vi "BuildHeaderData.vi"(5 "ScanFunc":i32, 6 "chemin Data":path, 8 "error in":errorcluster caption="entrée d'erreur (pas d'erreur)", 9 "SinglePar":bool, 10 "IndCourbe":i64, 11 "Experiment.lvclass In":refnum<class "Experiment.lvclass">) -> (0 "error out":errorcluster caption="sortie d'erreur", 1 "NomDon":string[](array[string])=["RTêta;", "X&Y;"], 2 "HeaderPar":string, 3 "Experiment.lvclass Out":refnum<class "Experiment.lvclass">, 4 "VarParams":string[][](array[string]), 7 "Experiment Name":string)   [LabVIEW 2019, in "Experiment.lvclass"]
uses:
  Experiment.lvclass
  Experiment.lvclass/Experiment.ctl
  DevicesClass/BaseDevice/BaseDevice.lvclass/BaseDevice.ctl
  DevicesClass/BaseDevice/Accessor/SetBaseDataPath.vi
  DevicesClass/BaseDevice/BaseDevice.lvclass
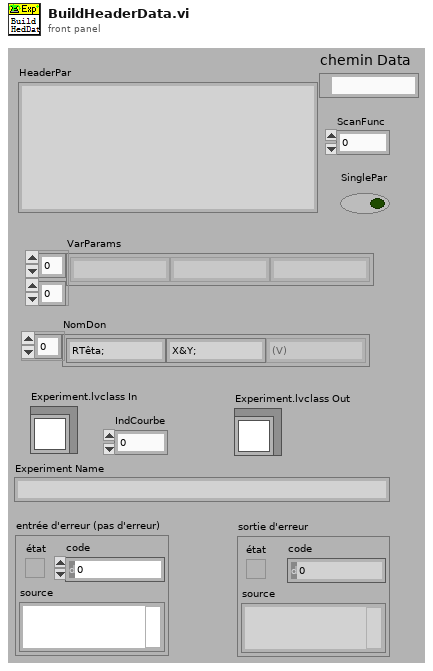
[diagram p1: front panel]
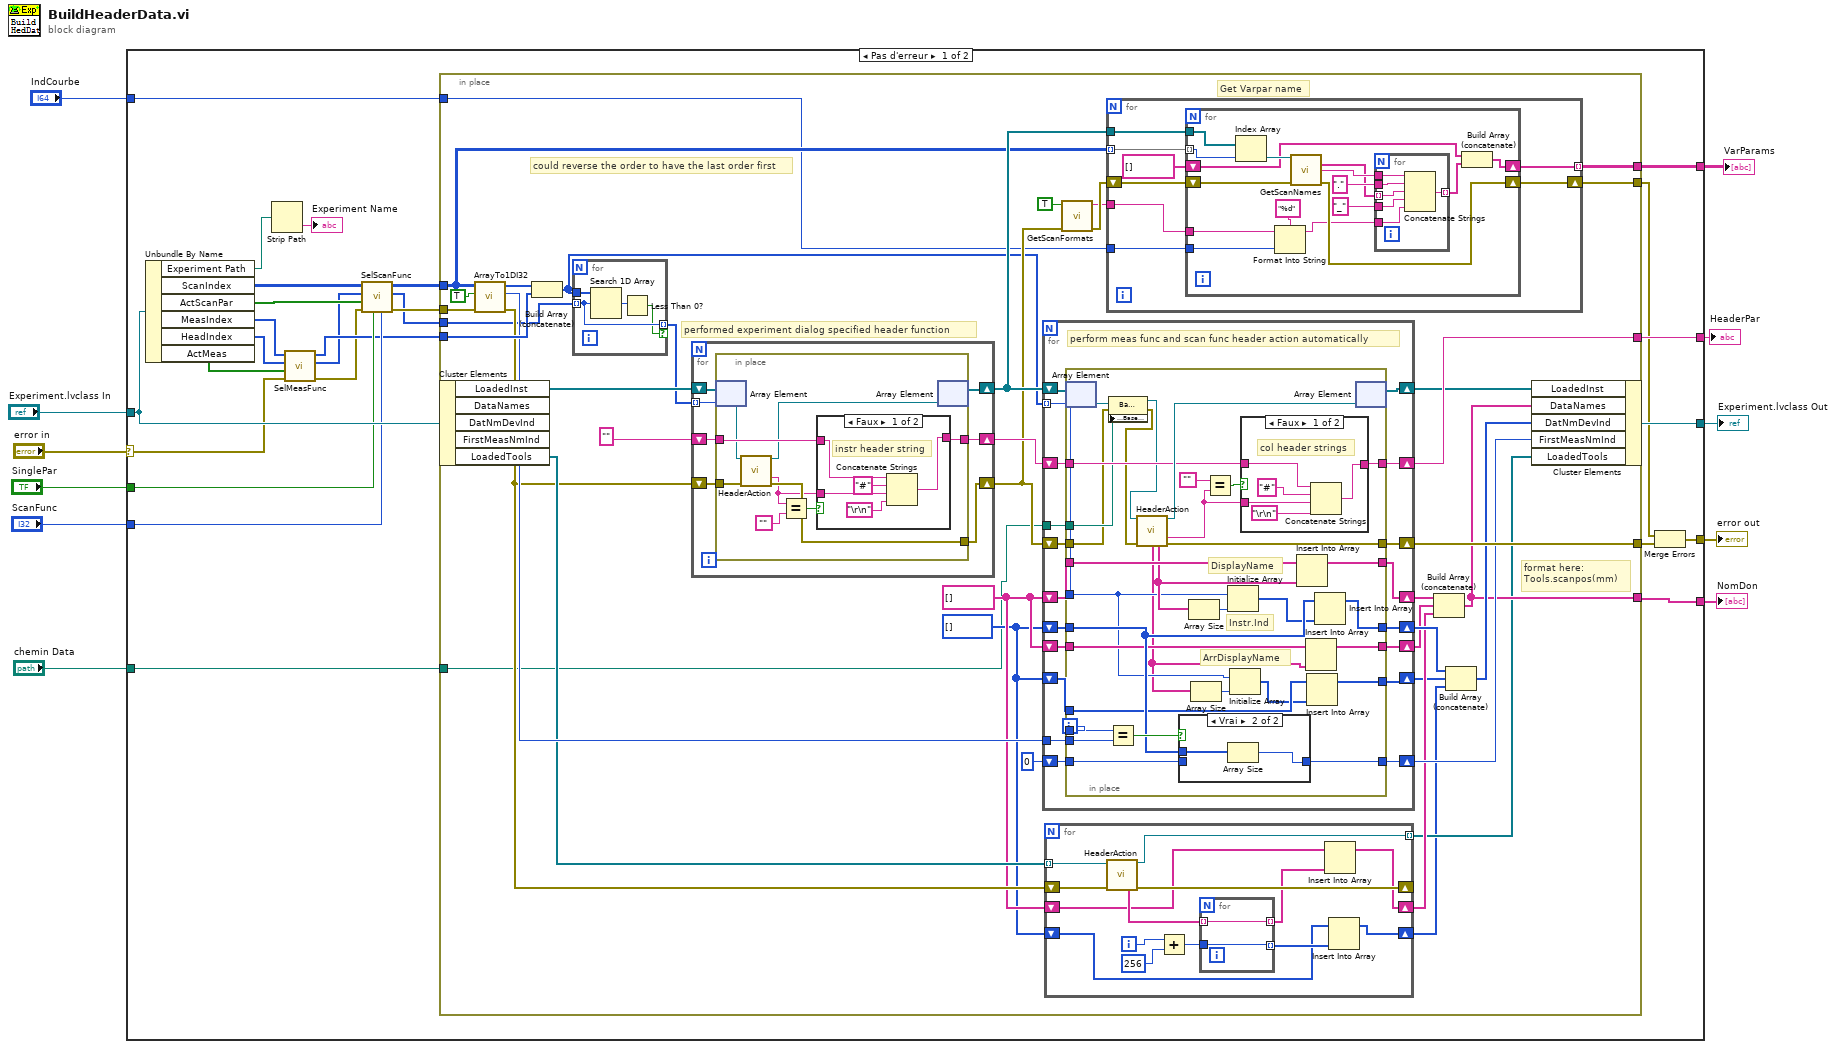
[diagram p0: block diagram]
diagram:
  n1 = case shown="Pas d'erreur" "error in" {
    selector: "error in" -> [w18 w211]
    tunnel: [w30 w211] -> w10
    tunnel: [w37 _] -> w9
    tunnel: [w33 _] -> w8
    tunnel: "Experiment.lvclass In" -> [w36 w210]
    tunnel: [w35 w210] -> w6
    tunnel: [w32 _] -> w5
    tunnel: "IndCourbe" -> [w31 _]
    tunnel: "SinglePar" -> [w20 _]
    tunnel: "ScanFunc" -> [w19 _]
    tunnel: "chemin Data" -> [w27 _]
    frame No Error {
      n2 = Unbundle By Name(w36) -> ("Experiment Path"=w21:path, "ScanIndex"=w23:i32[][], "ActScanPar"=w22:bool[], "MeasIndex"=w15:i32[], "HeadIndex"=w17:i32[], "ActMeas"=w14:bool[])
      n3 = Strip Path(path=w21) -> (name=→"Experiment Name":string)  [unwired: 1 out]
      n4 = call "SelMeasFunc.vi"("ErrorIn(No Error)"=w18, "Active MeasPar"=w14, "ScanHeaderIn"=w17, "MeasIndexIn"=w15) -> ("sortie d'erreur"=w13:errorcluster, "ScanHeaderOut"=w12:i32[], "MeasIndexOut"=w16:i32[])  [unwired: 5 in]
      n5 = call "SelScanFunc.vi"("Function"=w19, "SInglePar"=w20, "ErrorIn(No Error)"=w13, "Active ScanPar"=w22, "ScanHeaderIn"=w12, "ScanIndexIn"=w23) -> ("sortie d'erreur"=w26:errorcluster, "ScanHeaderOut"=w24:i32[], "ScanIndexOut"=w25:i32[][])  [unwired: 3 in]
      n6 = in-place {
        in-place-border: [w76] -> w37
        in-place-border: [w49] -> w33
        in-place-border: w26 -> [w71]
        in-place-border: w16 -> [w69]
        in-place-border: [w68] -> w34
        in-place-border: w25 -> [w61]
        in-place-border: w24 -> [w41]
        in-place-border: [w62] -> w32
        in-place-border: w31 -> [w56]
        in-place-border: [w55] -> w29
        in-place-border: w27 -> [w38]
        w45 = i32[] []
        w46 = string[] []
        # "format here:\nTools.scanpos(mm)"
        # "performed experiment dialog specified header function"
        # "Get Varpar name"
        # "could reverse the order to have the last order first"
        n7 = in-place-cluster #1(w36) -> ("LoadedInst"=w73:refnum<class "BaseDevice.lvclass">[], "LoadedTools"=w53:refnum<class "BaseDevice.lvclass">[])  [unwired: 3 out]
        n8 = call <userlib>:"ArrayTo1DI32.vi"("ErrorIn(No Error)"=w71, "DelArrEnd"=TRUE, "tableau"=w61) -> ("sortie d'erreur"=w52:errorcluster, "Size"=w66:i32, "Array Out"=w70:i32[])  [unwired: 6 in]
        n9 = Build Array (concatenate)(w70, w69) -> (w40:i32[])
        n10 = for {
          tunnel: w41 -> [w78] mode=indexing
          tunnel: w40 -> [w80]
          tunnel: [w78] -> w39 mode=indexing if=w77
          n11 = Search 1D Array(1D array=w80, element=w78) -> (index of element=w79:i32)  [unwired: 1 in]
          n12 = Less Than 0?(x=w79) -> (x < 0?=w77:bool)
        }
        n13 = for {
          shift-right: [w131] -> w74
          shift-left: "" -> [w132]
          tunnel: w39 -> [w130] mode=indexing
          shift-right: [w128] -> w63
          shift-left: w73 -> [w129]
          shift-right: [w127] -> w58
          shift-left: w52 -> [w133]
          n14 = in-place {
            in-place-border: w133 -> [w142]
            in-place-border: w132 -> [w141]
            in-place-border: [w138] -> w127
            in-place-border: [w136] -> w131
            n15 = in-place-array #2(w129, w130) -> (w135:refnum<class "BaseDevice.lvclass">)
            n16 = call-dynamic "HeaderAction.vi"("Device en entrée"=w135, "error in (no error)"=w142) -> ("Device en sortie"=w134:refnum<class "BaseDevice.lvclass">, "HeaderString"=w137:string, "error out"=w138:errorcluster)  [unwired: 7 in, 4 out]
            n17 = Equal?(x=w137, y="") -> (x = y?=w140:bool)
            n18 = case shown="Faux" w140 {
              tunnel: [w146 w148] -> w136
              tunnel: w137 -> [w144 _]
              tunnel: w141 -> [w145 w148]
              frame False {
                # "instr header string"
                n19 = Concatenate Strings(w145, "#" ("chaîne"), w144, "\r\n") -> (w146:string)
              }
              frame True {
              }
            }
            n20 = in-place-array #2(w134) -> (w128:refnum<class "BaseDevice.lvclass">[])  [unwired: 1 out]
          }
        }
        n21 = for {
          shift-right: [w167] -> w76
          shift-left: w74 -> [w164]
          shift-right: [w166] -> w50
          shift-left: w46 -> [w165]
          tunnel: w40 -> [w160] mode=indexing
          shift-right: [w162] -> w72
          shift-left: w63 -> [w163]
          shift-right: [w161] -> w68
          shift-left: w58 -> [w168]
          shift-right: [w159] -> w67
          shift-left: w45 -> [w158]
          tunnel: w66 -> [w157]
          shift-right: [w155] -> w64
          shift-left: 0 -> [w154]
          shift-right: [w153] -> w42
          shift-left: w46 -> [w152]
          shift-right: [w150] -> w43
          shift-left: w45 -> [w151]
          tunnel: w38 -> [w149]
          i -> [w156]
          # "perform meas func and scan func header action automatically"
          n22 = in-place {
            in-place-border: w168 -> [w170]
            in-place-border: [w200] -> w161
            in-place-border: [w199] -> w167
            in-place-border: [w198] -> w166
            in-place-border: w165 -> [w197]
            in-place-border: w164 -> [w192]
            in-place-border: w160 -> [w177]
            in-place-border: [w190] -> w159
            in-place-border: w158 -> [w186]
            in-place-border: w157 -> [w188]
            in-place-border: w156 -> [w189]
            in-place-border: [w185] -> w155
            in-place-border: w154 -> [w184]
            in-place-border: [w179] -> w153
            in-place-border: w152 -> [w178]
            in-place-border: w151 -> [w176]
            in-place-border: [w174] -> w150
            in-place-border: w149 -> [w172]
            # "ArrDisplayName"
            # "Instr.Ind"
            # "DisplayName"
            n23 = in-place-array #3(w163, w160) -> (w191:refnum<class "BaseDevice.lvclass">)
            n24 = Equal?(x=w189, y=w188) -> (x = y?=w187:bool)
            n25 = property class="BaseDevice.lvclass"(reference=w191, error in=w170, "Accessor:BaseDataPath"=w172) -> (reference out=w171:refnum<class "BaseDevice.lvclass">, error out=w169:errorcluster)
            n26 = call-dynamic "HeaderAction.vi"("Device en entrée"=w171, "error in (no error)"=w169) -> ("Device en sortie"=w193:refnum<class "BaseDevice.lvclass">, "HeaderString"=w196:string, "ArrDatNames"=w173:string[], "DisplayNames"=w180:string[], "error out"=w200:errorcluster)  [unwired: 7 in, 2 out]
            n27 = case shown="Vrai" w187 {
              tunnel: w186 -> [_ w203]
              tunnel: [w201 w202] -> w185
              tunnel: w184 -> [w201 _]
              frame False {
              }
              frame True {
                n28 = Array Size(array=w203) -> (size(s)=w202:i32)
              }
            }
            n29 = Array Size(array=w180) -> (size(s)=w182:i32)
            n30 = Array Size(array=w173) -> (size(s)=w181:i32)
            n31 = Equal?(x="", y=w196) -> (x = y?=w194:bool)
            n32 = Initialize Array(w177, w182) -> (w183:i32[])
            n33 = Initialize Array(w177, w181) -> (w175:i32[])
            n34 = case shown="Faux" w194 {
              tunnel: [w204 w209] -> w199
              tunnel: w196 -> [w208 _]
              tunnel: w192 -> [w205 w209]
              frame False {
                # "col header strings"
                n35 = Concatenate Strings(w205, "#" ("chaîne"), w208, "\r\n") -> (w204:string)
              }
              frame True {
              }
            }
            n36 = Insert Into Array(array=w197, new element=w180) -> (w198:string[])  [unwired: 1 in]
            n37 = Insert Into Array(array=w178, new element=w173) -> (w179:string[])  [unwired: 1 in]
            n38 = Insert Into Array(array=w176, new element=w175) -> (w174:i32[])  [unwired: 1 in]
            n39 = Insert Into Array(array=w186, new element=w183) -> (w190:i32[])  [unwired: 1 in]
            n40 = in-place-array #3(w193) -> (w162:refnum<class "BaseDevice.lvclass">[])  [unwired: 1 out]
          }
        }
        n41 = for {
          tunnel: w53 -> [w94] mode=indexing
          shift-right: [w92] -> _
          shift-left: w52 -> [w93]
          shift-right: [w84] -> w48
          shift-left: w46 -> [w86]
          shift-right: [w89] -> w44
          shift-left: w45 -> [w88]
          tunnel: [w81] -> w47 mode=indexing
          i -> [w87]
          n42 = call-dynamic "HeaderAction.vi"("Device en entrée"=w94, "error in (no error)"=w93) -> ("Device en sortie"=w81:refnum<class "BaseDevice.lvclass">, "DisplayNames"=w91:string[], "error out"=w92:errorcluster)  [unwired: 7 in, 4 out]
          n43 = Add(x=w87, y=256) -> (x+y=w83:i32)
          n44 = for {
            tunnel: [w95] -> w85 mode=indexing
            tunnel: w83 -> [w96]
            tunnel: [w96] -> w90 mode=indexing
            tunnel: w91 -> [w95] mode=indexing
          }
          n45 = Insert Into Array(array=w86, new element=w85) -> (w84:string[])  [unwired: 1 in]
          n46 = Insert Into Array(array=w88, new element=w90) -> (w89:i32[])  [unwired: 1 in]
        }
        n47 = call "GetScanFormats.vi"("ErrorIn(No Error)"=w58, "Scan(T)"=TRUE) -> ("sortie d'erreur"=w59:errorcluster, "Prefixe"=w57:string)  [unwired: 7 in, 1 out]
        n48 = for {
          tunnel: w61 -> [w104] mode=indexing
          shift-right: [w99] -> w55
          shift-left: w59 -> [w102]
          tunnel: [w100] -> w62 mode=indexing
          tunnel: w63 -> [w103]
          tunnel: w57 -> [w98]
          tunnel: w56 -> [w97]
          n49 = for {
            tunnel: w104 -> [w119] mode=indexing
            tunnel: w103 -> [w120]
            shift-right: [w113] -> w99
            shift-left: w102 -> [w114]
            shift-right: [w110] -> w100
            shift-left: string[] [] -> [w112]
            tunnel: w98 -> [w108]
            tunnel: w97 -> [w105]
            n50 = Index Array(array=w120, index=w119) -> (element=w118:refnum<class "BaseDevice.lvclass">)
            n51 = Format Into String(format string="%d" ("chaîne de format"), initial string=w108, w105) -> (resulting string=w106:string)  [unwired: 1 in, 1 out]
            n52 = call "GetScanNames.vi"("BaseDevice en entrée"=w118, "error in (no error)"=w114) -> ("DataNames"=w115:string[], "Instr Name"=w116:string, "error out"=w113:errorcluster)  [unwired: 10 in, 1 out]
            n53 = for {
              tunnel: w115 -> [w126] mode=indexing
              tunnel: "." ("chaîne") -> [w125]
              tunnel: [w124] -> w111 mode=indexing
              tunnel: w116 -> [w123]
              tunnel: "_" ("chaîne") -> [w122]
              tunnel: w106 -> [w121]
              n54 = Concatenate Strings(w123, w125, w126, w122, w121) -> (w124:string)
            }
            n55 = Build Array (concatenate)(w112, w111) -> (w110:string[])
          }
        }
        n56 = Build Array (concatenate)(w50, w42, w48) -> (w49:string[])
        n57 = Build Array (concatenate)(w67, w43, w44) -> (w51:i32[])
        n58 = in-place-cluster #1("LoadedInst"=w72, "DataNames"=w49, "DatNmDevInd"=w51, "FirstMeasNmInd"=w64, "LoadedTools"=w47) -> (w35:refnum<class "Experiment.lvclass">)
      }
      n59 = Merge Errors(w29, w34) -> (w30:errorcluster)
    }
    frame Error {
    }
  }
  "error out" <- w10
  "HeaderPar" <- w9
  "NomDon" <- w8
  "Experiment.lvclass Out" <- w6
  "VarParams" <- w5
